vi "Run.vi"(7 "Team Index":i32, 8 "Column":i32, 9 "Row":i32, 10 "View":i32[](array[numeric]) caption="View (Team Index, -1: empty)", 11 "Atomic In":refnum<class "Atomic.lvclass">) -> (0 "Replicated":refnum<class "Square.lvclass">, 1 "Direction":T1, 2 "Action":T2, 3 "Square Out":refnum<class "Square.lvclass">)   [LabVIEW 2017, in "Atomic.lvclass"]
uses:
  Atomic.lvclass
  SubVIs/SB SubVIs.lvlib
  GameMapData.ctl
  C:/Workspace/Endigit/SquareBattle/Square/Square.lvclass
  Square/Square.lvclass
  Type Defs/Action Enum.ctl
  Type Defs/SB Type Defs.lvlib
  Type Defs/Direction Enum.ctl
panel:
  # "NW\nN\nNE\nE\nSE\nS\nSW\nW"
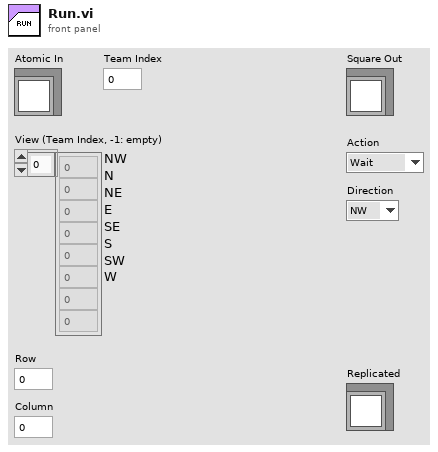
[diagram p1: front panel]
types:
  T1 = typedef "SB Type Defs.lvlib/Direction Enum.ctl" = enum16{"NW", "N", "NE", "E", "SE", "S", "SW", "W"}
  T2 = typedef "SB Type Defs.lvlib/Action Enum.ctl" = enum16{"Wait", "Move", "Attack", "Replicate"}
  T3 = typedef "GameMapData.ctl" = cluster{"View":i32[], "Data Age":i32, "Deaths":i32, "Victories":i32, "Plan":i16}
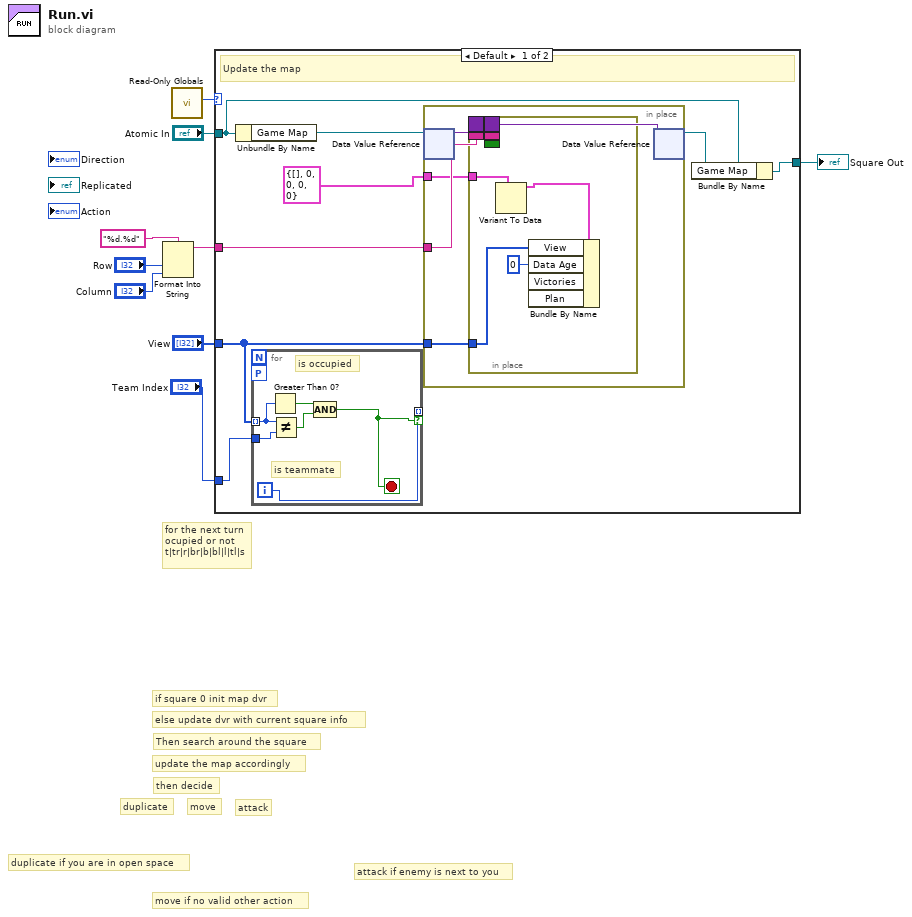
[diagram p0: block diagram]
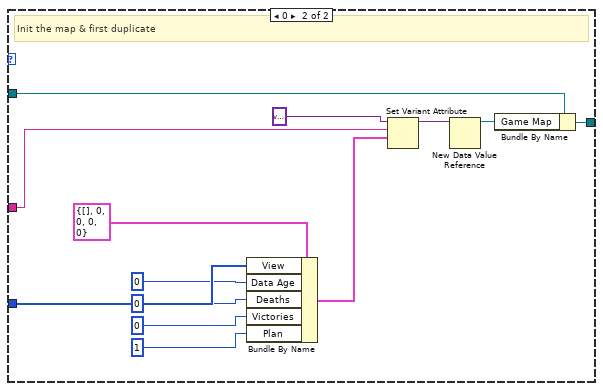
[diagram p2: hidden frame]
diagram:
  # "for the next turn\nocupied or not\nt|tr|r|br|b|bl|l|tl|s"
  # "duplicate if you are in open space"
  # "move if no valid other action"
  # "attack if enemy is next to you"
  # "then decide"
  # "update the map accordingly"
  # "Then search around the square"
  # "else update dvr with current square info"
  # "if square 0 init map dvr"
  # "attack"
  # "move"
  # "duplicate"
  n1 = Format Into String(format string="%d.%d", "Row", "Column") -> (resulting string=w1:string)  [unwired: 2 in, 1 out]
  n2 = call "Read-Only Globals.vi"() -> ("Round"=w9:i32)  [unwired: 10 in, 1 out]
  n3 = case shown="Default" w9 {
    tunnel: "Atomic In" -> [w14 w47]
    tunnel: "Team Index" -> [w10 _]
    tunnel: "View" -> [w11 w41]
    tunnel: [w12 w36] -> w3
    tunnel: w1 -> [w16 w35]
    frame Default {
      # "Update the map"
      n4 = Unbundle By Name(w14) -> ("Game Map"=w17:refnum<data-value>)
      n5 = for {
        tunnel: w11 -> [w22] mode=indexing
        tunnel: w10 -> [w23]
        workers-P: _ -> [_]
        tunnel: [w19] -> _ mode=indexing if=w18
        i -> [w19]
        stop <- w18 stop-if-true
        # "is occupied"
        # "is teammate"
        n6 = Greater Than 0?(x=w22) -> (x > 0?=w20:bool)
        n7 = Not Equal?(x=w22, y=w23) -> (x != y?=w21:bool)
        n8 = Compound Arithmetic op=AND(w20, w21) -> (w18:bool)
      }
      n9 = in-place {
        in-place-border: w16 -> [w27]
        in-place-border: T3 {"View"=[], "Data Age"=0, "Deaths"=0, "Victories"=0, "Plan"=0} ("value") -> [w25]
        in-place-border: w11 -> [w24]
        n10 = in-place-dvr #1(w17) -> (w28:variant)  [unwired: 1 out]
        n11 = in-place {
          border: w28 -> [_]
          border: w27 -> [_]
          border: [_] -> w26
          border: _ -> [_]
          border: _ -> [_]
          in-place-border: w25 -> [w34]
          in-place-border: w24 -> [w30]
          n12 = Variant To Data(type=w34, Variant=w33) -> (data=w32:T3)  [unwired: 1 in, 1 out]
          n13 = Bundle By Name(cluster=w32, "View"=w30, "Data Age"=0) -> (w31:T3)  [unwired: 2 in]
        }
        n14 = in-place-dvr #1(w26) -> (w13:refnum<data-value>)  [unwired: 1 out]
      }
      n15 = Bundle By Name(cluster=w14, "Game Map"=w13) -> (w12:refnum<class "Atomic.lvclass">)
    }
    frame 0 {
      # "Init the map & first duplicate"
      n16 = Bundle By Name(cluster=T3 {"View"=[], "Data Age"=0, "Deaths"=0, "Victories"=0, "Plan"=0} ("value"), "View"=w41, "Data Age"=0, "Deaths"=0, "Victories"=0, "Plan"=i16 1) -> (w44:T3)
      n17 = Set Variant Attribute(Variant=variant ("variant"), name=w35, value=w44) -> (Variant out=w46:variant)  [unwired: 1 in, 2 out]
      n18 = New Data Value Reference(data value=w46) -> (data value reference=w45:refnum<data-value>)  [unwired: 1 in, 1 out]
      n19 = Bundle By Name(cluster=w47, "Game Map"=w45) -> (w36:refnum<class "Atomic.lvclass">)
    }
  }
  "Square Out" <- w3
